vi "Relay_OFF.vi"(8 "error in (no error)":errorcluster, 11 "IN":T1={"step name 1"="", "updata 2"="1000", "limitdata 3"="", "load vi name 4"="", "parameter 5"=""}) -> (0 "error out":errorcluster, 3 "Cluster":T2)   [LabVIEW 2013]
uses:
  SubVi/Global constant.vi
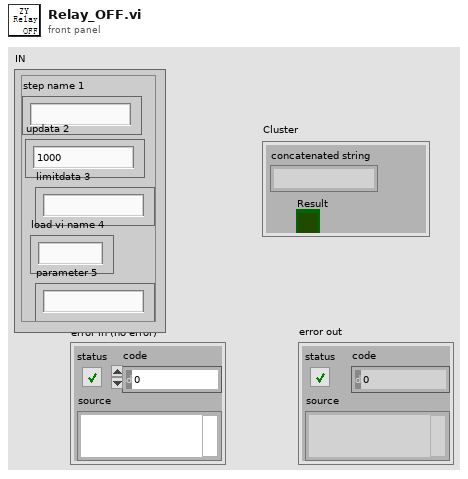
[diagram p1: front panel]
types:
  T1 = cluster{"step name 1":string, "updata 2":string, "limitdata 3":string, "load vi name 4":string, "parameter 5":string}
  T2 = cluster{"concatenated string":string, "Result":bool}
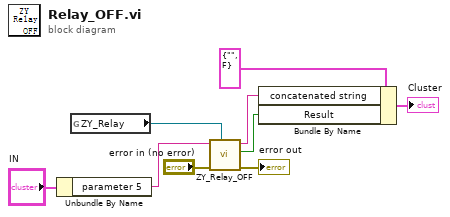
[diagram p0: block diagram]
diagram:
  n1 = Unbundle By Name("IN") -> ("parameter 5"=w1:string)
  n2 = global read "Global constant.vi" "ZY_Relay"() -> (w2:refnum<visa-resource-name>)
  n3 = call "ZY_Relay_OFF.vi"("COM"=w2, "error in (no error)"="error in (no error)", "Limit in"=w1) -> ("error out"=→"error out":errorcluster, "Result"=w4:bool, "String"=w3:string)  [unwired: 6 in]
  n4 = Bundle By Name(cluster=T2 {"concatenated string"="", "Result"=FALSE} ("Cluster"), "concatenated string"=w3, "Result"=w4) -> (→"Cluster":T2)
